vi "Steering_converter.vi"(6 "Yaw":dbl, 9 "setpoint":dbl, 10 "output":dbl, 11 "Degree allowence":dbl) -> (3 "Steer":dbl)   [LabVIEW 2017]
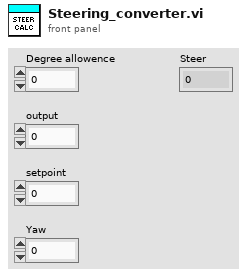
[diagram p1: front panel]
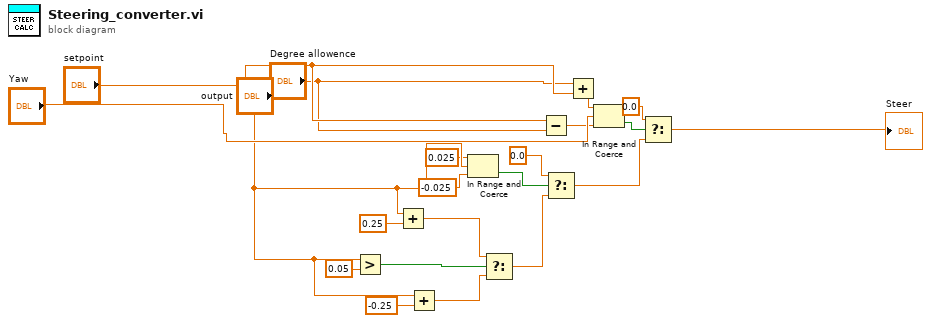
[diagram p0: block diagram]
diagram:
  n1 = Greater?(x="output", y=0.05) -> (0:w10:bool)
  n2 = Add(x="output", y=0.25) -> (x+y=w13:dbl)
  n3 = Add(x="output", y=-0.25) -> (x+y=w14:dbl)
  n4 = In Range and Coerce(upper limit=0.025, x="output", lower limit=-0.025) -> (In Range?=w9:bool)  [unwired: 1 out]
  n5 = Select(t=w13, s=w10, f=w14) -> (s? t:f=w16:dbl)
  n6 = Subtract(x="setpoint", y="Degree allowence") -> (x-y=w1:dbl)
  n7 = Select(t=0.0, s=w9, f=w16) -> (s? t:f=w17:dbl)
  n8 = Add(x="Degree allowence", y="setpoint") -> (x+y=w3:dbl)
  n9 = In Range and Coerce(upper limit=w3, x="Yaw", lower limit=w1) -> (In Range?=w4:bool)  [unwired: 1 out]
  n10 = Select(t=0.0, s=w4, f=w17) -> (s? t:f=→"Steer":dbl)
